vi "QTrkGetZLUT.vi"(8 "error in (no error)":errorcluster, 11 "QTrk Instance (in)":T1={"QTrk Pointer"=0, "QTrk Settings"={"Image width"=150, "Image height"=150, "Number of threads (CPU based)"=-1, "Max Queue Size"=128, "XCOR Profile Length"=32, "XCOR Profile Width"=2, "XCOR Iterations"=5, "ZLUT MinRadius"=50.0, "ZLUT MaxRadius"=64.0, "ZLUT AngularSteps"=0, "QI Iterations"=64, "QI RadialSteps"=64, "QI AngularSteps Per Quadrant"=2, "QI MinRadius"=50.0, "QI MaxRadius"=50.0, "CUDA Device# (if using cuda)"=0, "COM Background correction factor"=2.0, "ZLUT RadialSteps"=32, "Gaussian 2D Fit Iterations"=8}}) -> (0 "error out":errorcluster, 2 "zlut":sgl[][][](array[numeric]), 3 "QTrk Instance":T1={"QTrk Pointer"=0, "QTrk Settings"={"Image width"=150, "Image height"=150, "Number of threads (CPU based)"=-1, "Max Queue Size"=128, "XCOR Profile Length"=32, "XCOR Profile Width"=2, "XCOR Iterations"=5, "ZLUT MinRadius"=50.0, "ZLUT MaxRadius"=64.0, "ZLUT AngularSteps"=0, "QI Iterations"=64, "QI RadialSteps"=64, "QI AngularSteps Per Quadrant"=2, "QI MinRadius"=50.0, "QI MaxRadius"=50.0, "CUDA Device# (if using cuda)"=0, "COM Background correction factor"=2.0, "ZLUT RadialSteps"=32, "Gaussian 2D Fit Iterations"=8}})   [LabVIEW 2011]
uses:
  QTrkInstance.ctl
  QTrkSettings.ctl
  QTrkDLL.vi
panel:
  in  "ZLUT":sgl[][][](array[numeric])
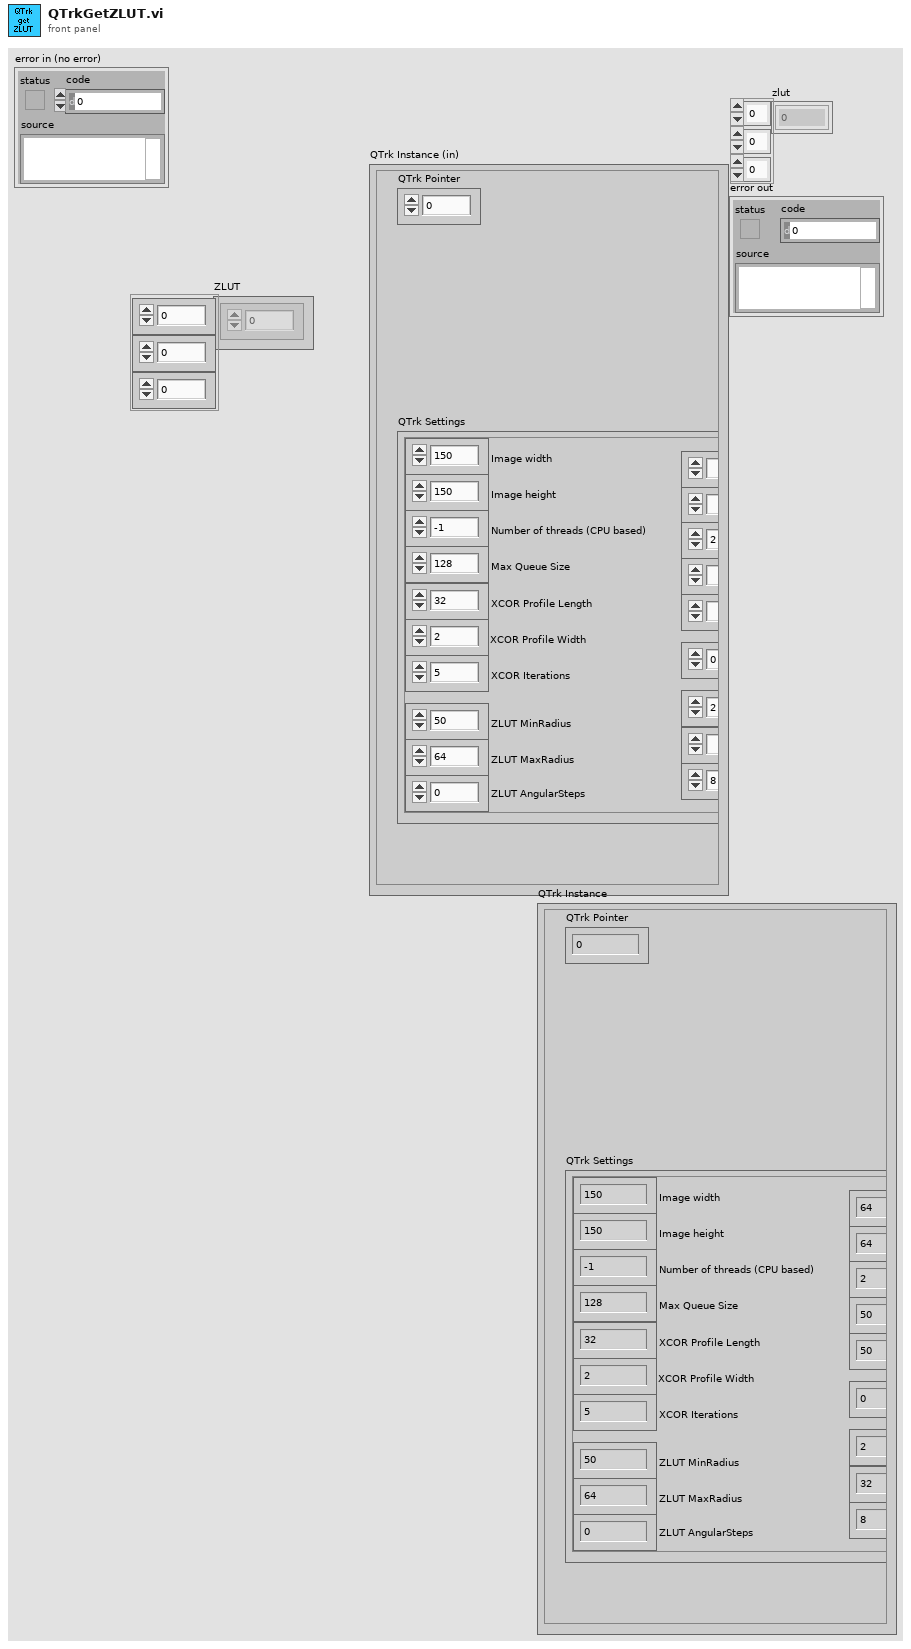
[diagram p1: front panel]
types:
  T1 = typedef "QTrkInstance.ctl" = cluster{"QTrk Pointer":u64, "QTrk Settings":T2}
  T2 = typedef "QTrkSettings.ctl" = cluster{"Image width":i32, "Image height":i32, "Number of threads (CPU based)":i32, "Max Queue Size":i32, "XCOR Profile Length":i32, "XCOR Profile Width":i32, "XCOR Iterations":i32, "ZLUT MinRadius":sgl, "ZLUT MaxRadius":sgl, "ZLUT AngularSteps":i32, "QI Iterations":i32, "QI RadialSteps":i32, "QI AngularSteps Per Quadrant":i32, "QI MinRadius":sgl, "QI MaxRadius":sgl, "CUDA Device# (if using cuda)":i32, "COM Background correction factor":sgl, "ZLUT RadialSteps":i32, "Gaussian 2D Fit Iterations":i32}
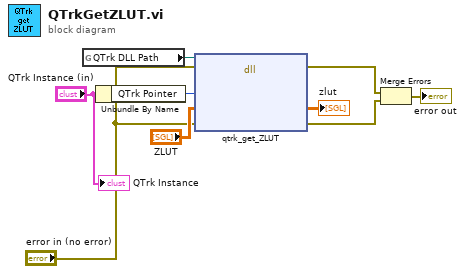
[diagram p0: block diagram]
diagram:
  n1 = global read "QTrkDLL.vi" "QTrk DLL Path"() -> (w6:path)
  n2 = Unbundle By Name("QTrk Instance (in)") -> ("QTrk Pointer"=w8:u64)
  n3 = dll-call lib="D:/jcnossen1/cudaqi-tracker/bin/jtrk-labview.dll" fn="qtrk_get_ZLUT"(path in=w6, error in="error in (no error)", "tracker"=w8, "zlut"="ZLUT", "error"="error in (no error)") -> (error out=w3:errorcluster, "zlut"=→"zlut":sgl[][][], "error"=w2:errorcluster)  [unwired: 3 in, 1 out]
  n4 = Merge Errors(w3, w2) -> (→"error out":errorcluster)
  "QTrk Instance" <- "QTrk Instance (in)"
